vi "Check Stream Status.vi"(0 "niUsrpRio Session":T1={"FPGA Interface"=refnum, "RIO Interface Number"=0, "Data Clock Rate"=0, "FPGA Data Clock Rate"=0, "Global Settings Register Bus"=refnum, "Radio 0 Settings Register Bus"=refnum, "Radio 1 Settings Register Bus"=refnum, "Radio Settings Bus Semaphore"=refnum, "DB Queues"=[], "Characterization Data Valid?"=FALSE, "EEPROM Header"={"Checksum"=0, "Product Code"=0, "Hardware Current Version"=0, "Hardware Oldest Compatible Version"=0, "EEPROM Map Current Version"=0, "EEPROM Map Oldest Compatible Version"=0, "User Password"="", "Pointer to Factory Header"=0, "Pointer to User Header"=0, "Recommended Interval"=0, "Number of Reserved Bytes"=9, "Number of Daughterboards"=0, "Daughterboard IDs"=[], "Daughterboard Serial Numbers"=[]}, "Device Data Header"={"Checksum"=0, "Number of Channels"=0, "Number of Gain Settings"=[], "Pointer to Characterization Data"=[], "Number of Reserved Bytes"=27, "Number of Frequencies"=[]}, "EEPROM Characterization Header"={"Checksum"=0, "Date"=timestamp(0 s since 1904-01-01), "Temperature"=0.0, "Misc. Info"="", "Pointer to Device Data Header"=0, "Number of Reserved Bytes"=28}, "Characterization Data"=[], "FPGA Current Version"=0, "FPGA Oldest Compatible Version"=0, "Fixed Logic Current Version"=0, "Fixed Logic Oldest Compatible Version"=0, "FPGA Radio Settings Bus Current Version"=0, "FPGA Radio Settings Bus Oldest Compatible Version"=0, "FPGA Board Config Current Version"=0, "FPGA Board Config Oldest Compatible Version"=0, "Daughterboard Clock Rate"=0, "daughterboard configuration session handles"=[]} {"Daughterboard Clock Rate" format="%#.3pHz"; "FPGA Data Clock Rate" format="%#.3pHz"; "Data Clock Rate" format="%#.3pHz"; "Characterization Data"."Frequencies [Hz]" format="%#_6p"; "EEPROM Characterization Header"."Pointer to Device Data Header" format="%x"; "EEPROM Characterization Header"."Checksum" format="%x"; "Device Data Header"."Pointer to Characterization Data" format="%x"; "Device Data Header"."Checksum" format="%x"; "EEPROM Header"."Pointer to User Header" format="%x"; "EEPROM Header"."Pointer to Factory Header" format="%x"; "EEPROM Header"."Product Code" format="%x"; "EEPROM Header"."Checksum" format="%x"}, 1 "scope":string(combo)="rx", 11 "error in":errorcluster, 12 "reference frequency source":string(combo)="Internal" caption="Reference Frequency Source") -> (4 "niUsrpRio Session (out)":T1={"FPGA Interface"=refnum, "RIO Interface Number"=0, "Data Clock Rate"=0, "FPGA Data Clock Rate"=0, "Global Settings Register Bus"=refnum, "Radio 0 Settings Register Bus"=refnum, "Radio 1 Settings Register Bus"=refnum, "Radio Settings Bus Semaphore"=refnum, "DB Queues"=[], "Characterization Data Valid?"=FALSE, "EEPROM Header"={"Checksum"=0, "Product Code"=0, "Hardware Current Version"=0, "Hardware Oldest Compatible Version"=0, "EEPROM Map Current Version"=0, "EEPROM Map Oldest Compatible Version"=0, "User Password"="", "Pointer to Factory Header"=0, "Pointer to User Header"=0, "Recommended Interval"=0, "Number of Reserved Bytes"=9, "Number of Daughterboards"=0, "Daughterboard IDs"=[], "Daughterboard Serial Numbers"=[]}, "Device Data Header"={"Checksum"=0, "Number of Channels"=0, "Number of Gain Settings"=[], "Pointer to Characterization Data"=[], "Number of Reserved Bytes"=27, "Number of Frequencies"=[]}, "EEPROM Characterization Header"={"Checksum"=0, "Date"=timestamp(0 s since 1904-01-01), "Temperature"=0.0, "Misc. Info"="", "Pointer to Device Data Header"=0, "Number of Reserved Bytes"=28}, "Characterization Data"=[], "FPGA Current Version"=0, "FPGA Oldest Compatible Version"=0, "Fixed Logic Current Version"=0, "Fixed Logic Oldest Compatible Version"=0, "FPGA Radio Settings Bus Current Version"=0, "FPGA Radio Settings Bus Oldest Compatible Version"=0, "FPGA Board Config Current Version"=0, "FPGA Board Config Oldest Compatible Version"=0, "Daughterboard Clock Rate"=0, "daughterboard configuration session handles"=[]} {"Daughterboard Clock Rate" format="%#.3pHz"; "FPGA Data Clock Rate" format="%#.3pHz"; "Data Clock Rate" format="%#.3pHz"; "Characterization Data"."Frequencies [Hz]" format="%#_6p"; "EEPROM Characterization Header"."Pointer to Device Data Header" format="%x"; "EEPROM Characterization Header"."Checksum" format="%x"; "Device Data Header"."Pointer to Characterization Data" format="%x"; "Device Data Header"."Checksum" format="%x"; "EEPROM Header"."Pointer to User Header" format="%x"; "EEPROM Header"."Pointer to Factory Header" format="%x"; "EEPROM Header"."Product Code" format="%x"; "EEPROM Header"."Checksum" format="%x"}, 6 "done":bool caption="Done", 15 "error out":errorcluster)   [LabVIEW 2021]
doc: "Checks the status of the stream for when it is done, for FIFO overflows, for FIFO underflows, for DSP overflows, and if the clocks ever became unlocked. Checks the stream status after each Fetch Rx Data/Write Tx Data.\n\n<B>Input Parameters</B>\n\n<B>niUsrpRio Session</B> is the object created by the Open VI and used as the session handle for the USRP RIO design library.\n\n<B>Reference Frequency Source</B> is used when the source is GPS to determine whether to check whether the GPS became unlocked.\n\n<B>scope</B> is the channel to check the stream status. The options are \"rx/RF 0\", \"rx/RF 1\", \"tx/RF 0\", and \"tx/RF 1\".\n\n<B>error in</B> describes error conditions that occur before this node runs. This input provides standard 'error in' functionality.\n\n<B>Output Parameters</B>\n\n<B>niUsrpRio Session (out)</B> is the niUsrpRio session used in all subsequent USRP RIO design library host VIs.\n\n<B>Done</B> indicates when the acquisition/generation has completed.\n\n<B>error out</B> contains error information. This output provides standard 'error out' functionality."
uses:
  <instrlib>/niUsrpRio/Config/v1/Host/Public/niUsrpRio Session.ctl
  <instrlib>/_niInstr/Register Bus/v0/Host/Public/Register Bus Session.ctl
  <instrlib>/_niInstr/Register Bus/v0/Host/Private/Session Data.ctl
  <instrlib>/niUsrpRio/Config/v1/Host/Private/DB Queue Reference.ctl
  <instrlib>/niUsrpRio/Config/v1/Host/Private/Daughterboard Data.ctl
  <instrlib>/niUsrpRio/Config/v1/Host/Private/ATR state data.ctl
  <instrlib>/niUsrpRio/Config/v1/Host/Private/Antenna Configuration.ctl
  <instrlib>/niUsrpRio/Config/v1/Host/Private/CPLD Power Mode.ctl
  <instrlib>/niUsrpRio/Config/v1/Host/Public/EEPROM Header.ctl
  <instrlib>/niUsrpRio/Config/v1/Host/Public/EEPROM Device Data Header.ctl
  <instrlib>/niUsrpRio/Config/v1/Host/Public/EEPROM Characterization Header.ctl
  <instrlib>/niUsrpRio/Config/v1/Host/Public/Characterization Data.ctl
  <instrlib>/niUsrpRio/Config/v1/Host/Public/IQ Imbalance.ctl
  FPGA/SubVIs/Stream Control State.ctl
  Streaming Xvcr FPGA Ref.ctl
  <instrlib>/niUsrpRio/Config/v1/Host/Public/What to Query for.ctl
  <vilib>/rvi/errors/niLvFpgaAdjustHostInterfaceError.vi
  <vilib>/rvi/interface/nirviReadWriteControl/nirviReadWriteControl.xnode
  NiFpgaLv.dll
  <vilib>/rvi/interface/Simulation/niFpgaSimulationCallBeginRW.vi
  <instrlib>/niUsrpRio/Config/v1/Host/niUsrpRio Config v1 Host.lvlib
  <instrlib>/_niInstr/Register Bus/v0/Host/niInstr Register Bus v0 Host.lvlib
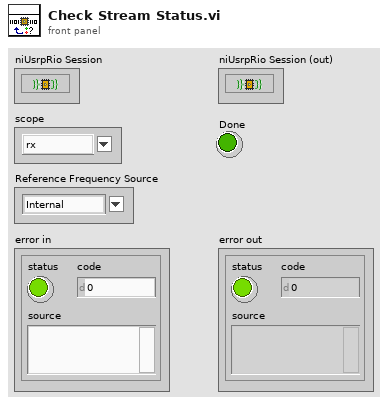
[diagram p1: front panel]
types:
  T1 = typedef "niUsrpRio Config v1 Host.lvlib/niUsrpRio Session.ctl" = cluster{"FPGA Interface":refnum<k20>, "RIO Interface Number":u32, "Data Clock Rate":u32, "FPGA Data Clock Rate":u32, "Global Settings Register Bus":T2, "Radio 0 Settings Register Bus":T2, "Radio 1 Settings Register Bus":T2, "Radio Settings Bus Semaphore":T3, "DB Queues":T4[], "Characterization Data Valid?":bool, "EEPROM Header":T5, "Device Data Header":T6, "EEPROM Characterization Header":T7, "Characterization Data":T8[], "FPGA Current Version":u32, "FPGA Oldest Compatible Version":u32, "Fixed Logic Current Version":u32, "Fixed Logic Oldest Compatible Version":u32, "FPGA Radio Settings Bus Current Version":u32, "FPGA Radio Settings Bus Oldest Compatible Version":u32, "FPGA Board Config Current Version":u32, "FPGA Board Config Oldest Compatible Version":u32, "Daughterboard Clock Rate":u32, "daughterboard configuration session handles":u64[]}
  T2 = typedef "niInstr Register Bus v0 Host.lvlib/Register Bus Session.ctl" = refnum<queue>
  T3 = typedef "Semaphore RefNum" = refnum<k1>
  T4 = typedef "niUsrpRio Config v1 Host.lvlib/DB Queue Reference.ctl" = refnum<queue>
  T5 = typedef "niUsrpRio Config v1 Host.lvlib/EEPROM Header.ctl" = cluster{"Checksum":u32, "Product Code":u16, "Hardware Current Version":u16, "Hardware Oldest Compatible Version":u16, "EEPROM Map Current Version":u16, "EEPROM Map Oldest Compatible Version":u16, "User Password":string, "Pointer to Factory Header":u32, "Pointer to User Header":u32, "Recommended Interval":u16, "Number of Reserved Bytes":i32, "Number of Daughterboards":u8, "Daughterboard IDs":u16[], "Daughterboard Serial Numbers":string[]}
  T6 = typedef "niUsrpRio Config v1 Host.lvlib/EEPROM Device Data Header.ctl" = cluster{"Checksum":u32, "Number of Channels":u8, "Number of Gain Settings":u16[], "Pointer to Characterization Data":u32[], "Number of Reserved Bytes":i32, "Number of Frequencies":u16[]}
  T7 = typedef "niUsrpRio Config v1 Host.lvlib/EEPROM Characterization Header.ctl" = cluster{"Checksum":u32, "Date":timestamp, "Temperature":sgl, "Misc. Info":string, "Pointer to Device Data Header":u32, "Number of Reserved Bytes":i32}
  T8 = typedef "niUsrpRio Config v1 Host.lvlib/Characterization Data.ctl" = cluster{"Gains[dB]":dbl[], "Frequencies [Hz]":dbl[], "IQ Imbalance Table":T9[], "Measured Gains[dB]":dbl[][]}
  T9 = typedef "niUsrpRio Config v1 Host.lvlib/IQ Imbalance.ctl" = cluster{"Gain Imbalance [linear]":dbl, "Phase Imbalance [radians]":dbl, "Offset":cdb}
  T10 = typedef "niUsrpRio Config v1 Host.lvlib/What to Query for.ctl" = enum16{"Clock Chip Lock Status", "Clock Chip Ever Unlocked", "LO Lock Status", "GPS Lock Status", "GPS Ever Unlocked", "DRAM Ready Status", "DAC PLL Lock Status", "DAC Sync Lock Status", "Data Clock PLL Lock Status", "Data Clock PLL Ever Unlocked", "ADC Clock PLL Lock Status", "ADC Clock PLL Ever Unlocked", "ADC Data Valid Status", "ADC Data Ever Invalid"}
  T11 = typedef "Streaming Xvcr FPGA Ref.ctl" = refnum<k20>
  T12 = typedef "Stream Control State.ctl" = enum16{"Idle", "Active"}
  T13 = typedef "niUsrpRio Config v1 Host.lvlib/Device Subfunction.ctl" = enum16{"rx", "tx", "all"}
  T14 = typedef "niUsrpRio Config v1 Host.lvlib/RF Channel 2.ctl" = enum16{"0", "1", "2", "3", "All"}
  T15 = typedef "niUsrpRio Config v1 Host.lvlib/DB Types.ctl" = enum16{"sbx", "cbx", "wbx", "unknown", "ubx", "twinrx"}
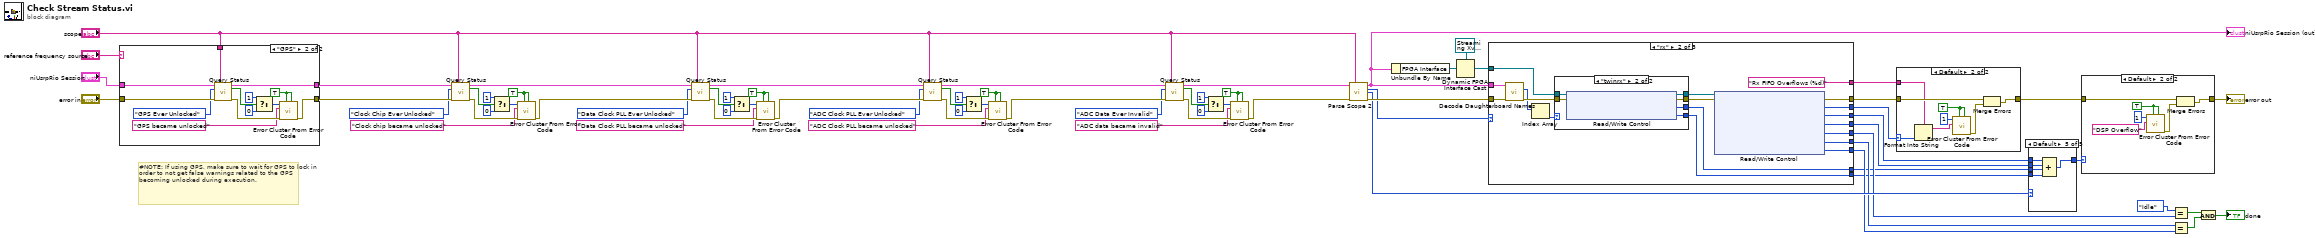
[diagram p0: block diagram]
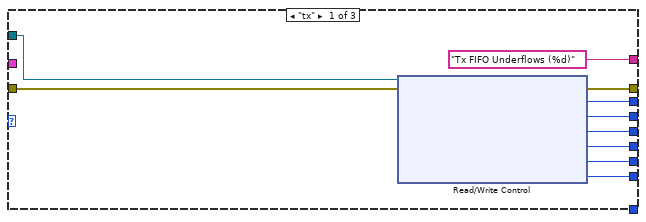
[diagram p9: hidden frame]
diagram:
  w15 = TRUE ("show call chain? (False)")
  w24 = TRUE ("show call chain? (False)")
  w29 = TRUE ("show call chain? (False)")
  w38 = TRUE ("show call chain? (False)")
  # "#NOTE: If using GPS, make sure to wait for GPS to lock in order to not get false warnings related to the GPS becoming unlocked during execution."
  n1 = case shown="\"GPS\"" "reference frequency source" {
    tunnel: "error in" -> [w71 w85]
    tunnel: "scope" -> [_ w73]
    tunnel: "niUsrpRio Session" -> [w72 w76]
    tunnel: [w72 w75] -> w10
    tunnel: [w71 w74] -> w70
    frame Default {
    }
    frame "GPS" {
      w81 = TRUE ("show call chain? (False)")
      n2 = call <instrlib>:"Query Status.vi"("niUsrpRio Session"=w76, "scope"=w73, "What to Query for"=What_to_Query_for."GPS Ever Unlocked", "error in"=w85) -> ("niUsrpRio Session (out)"=w75:T1, "Status"=w80:bool, "error out"=w84:errorcluster)  [unwired: 9 in]
      n3 = Select(t=1 ("error code (0)"), s=w80, f=0) -> (s? t:f=w79:i32)
      n4 = call <vilib>:"Error Cluster From Error Code.vi"("is warning? (False)"=w81, "show call chain? (False)"=w81, "error in (no error)"=w84, "error message (\"\")"="GPS became unlocked" ("error message (\"\")"), "error code (0)"=w79) -> ("error out"=w74:errorcluster)  [unwired: 4 in]
    }
  }
  n5 = call <instrlib>:"Query Status.vi"("niUsrpRio Session"=w10, "scope"="scope", "What to Query for"=What_to_Query_for."Clock Chip Ever Unlocked", "error in"=w70) -> ("niUsrpRio Session (out)"=w9:T1, "Status"=w37:bool, "error out"=w63:errorcluster)  [unwired: 9 in]
  n6 = Select(t=1 ("error code (0)"), s=w37, f=0) -> (s? t:f=w36:i32)
  n7 = call <vilib>:"Error Cluster From Error Code.vi"("is warning? (False)"=w38, "show call chain? (False)"=w38, "error in (no error)"=w63, "error message (\"\")"="Clock chip became unlocked" ("error message (\"\")"), "error code (0)"=w36) -> ("error out"=w69:errorcluster)  [unwired: 4 in]
  n8 = call <instrlib>:"Query Status.vi"("niUsrpRio Session"=w9, "scope"="scope", "What to Query for"=What_to_Query_for."Data Clock PLL Ever Unlocked", "error in"=w69) -> ("niUsrpRio Session (out)"=w8:T1, "Status"=w30:bool, "error out"=w66:errorcluster)  [unwired: 9 in]
  n9 = Select(t=1 ("error code (0)"), s=w30, f=0) -> (s? t:f=w31:i32)
  n10 = call <vilib>:"Error Cluster From Error Code.vi"("is warning? (False)"=w29, "show call chain? (False)"=w29, "error in (no error)"=w66, "error message (\"\")"="Data Clock PLL became unlocked" ("error message (\"\")"), "error code (0)"=w31) -> ("error out"=w68:errorcluster)  [unwired: 4 in]
  n11 = call <instrlib>:"Query Status.vi"("niUsrpRio Session"=w8, "scope"="scope", "What to Query for"=What_to_Query_for."ADC Clock PLL Ever Unlocked", "error in"=w68) -> ("niUsrpRio Session (out)"=w7:T1, "Status"=w23:bool, "error out"=w65:errorcluster)  [unwired: 9 in]
  n12 = Select(t=1 ("error code (0)"), s=w23, f=0) -> (s? t:f=w22:i32)
  n13 = call <vilib>:"Error Cluster From Error Code.vi"("is warning? (False)"=w24, "show call chain? (False)"=w24, "error in (no error)"=w65, "error message (\"\")"="ADC Clock PLL became unlocked" ("error message (\"\")"), "error code (0)"=w22) -> ("error out"=w67:errorcluster)  [unwired: 4 in]
  n14 = call <instrlib>:"Query Status.vi"("niUsrpRio Session"=w7, "scope"="scope", "What to Query for"=What_to_Query_for."ADC Data Ever Invalid", "error in"=w67) -> ("niUsrpRio Session (out)"=w6:T1, "Status"=w16:bool, "error out"=w64:errorcluster)  [unwired: 9 in]
  n15 = Select(t=1 ("error code (0)"), s=w16, f=0) -> (s? t:f=w17:i32)
  n16 = call <vilib>:"Error Cluster From Error Code.vi"("is warning? (False)"=w15, "show call chain? (False)"=w15, "error in (no error)"=w64, "error message (\"\")"="ADC data became invalid" ("error message (\"\")"), "error code (0)"=w17) -> ("error out"=w5:errorcluster)  [unwired: 4 in]
  n17 = call <instrlib>:"Parse Scope 2.vi"("niUsrpRio Session"=w6, "scope"="scope", "error in"=w5) -> ("niUsrpRio Session (out)"=w3:T1, "Device Subfunction"=w58:T13, "Device Subfunction Channel"=w51:T14, "error out"=w62:errorcluster)  [unwired: 4 in, 5 out]
  "niUsrpRio Session (out)" <- w3
  n18 = Unbundle By Name(w3) -> ("FPGA Interface"=w43:refnum<k20>)
  n19 = Dynamic FPGA Interface Cast(Session In=T11 refnum ("USRP RIO Streaming Xcvr FPGA VI Reference"), Type=w43) -> (Session Out=w42:T11)
  n20 = case shown="\"rx\"" w58 {
    tunnel: w62 -> [w95 w104 w122]
    tunnel: [w94 w112 _] -> w56
    tunnel: [w93 w111 w122] -> w57
    tunnel: [w92 w110 _] -> w53
    tunnel: [w91 w109 _] -> w52
    tunnel: [w90 w108 _] -> w49
    tunnel: [w89 w107 _] -> w48
    tunnel: [w88 w106 _] -> w47
    tunnel: ["Tx FIFO Underflows (%d)" ("error message (\"\")") "Rx FIFO Overflows (%d)" ("error message (\"\")") _] -> w55
    tunnel: w42 -> [w86 w99 _]
    tunnel: w3 -> [_ w103 _]
    tunnel: [_ w97 _] -> w2
    tunnel: [_ w96 _] -> w1
    frame "tx" {
      n21 = xnode "Read/Write Control"("FPGA VI Reference In"=w86, "error in"=w95) -> ("error out"=w93:errorcluster, "tx.number of fifo underflows"=w94:u32, "tx 0.number of iq data overflows"=w92:u64, "tx 1.number of iq data overflows"=w91:u64, "tx.state"=w90:enum16{"Idle", "Active"}, "tx.samples processed"=w89:u32, "tx.samples to generate"=w88:u32)  [unwired: 1 out]
    }
    frame "rx" {
      n22 = call <instrlib>:"Decode Daughterboard Names.vi"("niUsrpRio Session"=w103, "error in"=w104) -> ("daughterboard names"=w102:T15[], "error out"=w113:errorcluster)  [unwired: 10 in, 2 out]
      n23 = Index Array(array=w102) -> (element=w100:T15)  [unwired: 1 in]
      n24 = case shown="\"twinrx\"" w100 {
        tunnel: w113 -> [w115 w121]
        tunnel: [w115 w120] -> w101
        tunnel: w99 -> [w114 w119]
        tunnel: [w114 w118] -> w98
        tunnel: [_ w117] -> w97
        tunnel: [_ w116] -> w96
        frame Default {
        }
        frame "twinrx" {
          n25 = xnode "Read/Write Control"("FPGA VI Reference In"=w119, "error in"=w121) -> ("FPGA VI Reference Out"=w118:T11, "error out"=w120:errorcluster, "rx 2.number of iq data overflows"=w117:u64, "rx 3.number of iq data overflows"=w116:u64)
        }
      }
      n26 = xnode "Read/Write Control"("FPGA VI Reference In"=w98, "error in"=w101) -> ("error out"=w111:errorcluster, "rx.number of fifo overflows"=w112:u32, "rx 0.number of iq data overflows"=w110:u64, "rx 1.number of iq data overflows"=w109:u64, "rx.state"=w108:enum16{"Idle", "Active"}, "rx.samples processed"=w107:u32, "rx.samples to acquire"=w106:u32)  [unwired: 1 out]
    }
    frame Default {
    }
  }
  n27 = case shown="Default" w56 {
    selector: w56 -> [_ w125]
    tunnel: w57 -> [w123 w130]
    tunnel: [w123 w128] -> w54
    tunnel: w55 -> [_ w124]
    frame 0 {
    }
    frame Default {
      w126 = TRUE ("show call chain? (False)")
      n28 = Format Into String(format string=w124, w125) -> (resulting string=w127:string)  [unwired: 2 in, 1 out]
      n29 = call <vilib>:"Error Cluster From Error Code.vi"("is warning? (False)"=w126, "show call chain? (False)"=w126, "error message (\"\")"=w127, "error code (0)"=1) -> ("error out"=w129:errorcluster)  [unwired: 5 in]
      n30 = Merge Errors(w130, w129) -> (w128:errorcluster)
    }
  }
  n31 = case shown="Default" w51 {
    tunnel: w53 -> [w132 _ _ _ w140]
    tunnel: w52 -> [_ w133 _ _ w139]
    tunnel: [w132 w133 w134 w135 w138] -> w50
    tunnel: w2 -> [_ _ w134 _ w137]
    tunnel: w1 -> [_ _ _ w135 w136]
    frame "0" {
    }
    frame "1" {
    }
    frame "2" {
    }
    frame "3" {
    }
    frame Default {
      n32 = Compound Arithmetic op=ADD(w140, w139, w137, w136) -> (w138:u64)
    }
  }
  n33 = case shown="Default" w50 {
    tunnel: w54 -> [w141 w145]
    tunnel: [w141 w143] -> w45
    frame 0 {
    }
    frame Default {
      w142 = TRUE ("show call chain? (False)")
      n34 = call <vilib>:"Error Cluster From Error Code.vi"("is warning? (False)"=w142, "show call chain? (False)"=w142, "error message (\"\")"="DSP Overflow" ("error message (\"\")"), "error code (0)"=1) -> ("error out"=w144:errorcluster)  [unwired: 5 in]
      n35 = Merge Errors(w145, w144) -> (w143:errorcluster)
    }
  }
  "error out" <- w45
  n36 = Equal?(x=Stream_Control_State."Idle" ("state"), y=w49) -> (x = y?=w61:bool)
  n37 = Equal?(x=w48, y=w47) -> (x = y?=w60:bool)
  n38 = And(x=w61, y=w60) -> (x .and. y?=→"done":bool)
